vi "ReferenceGenerator_L.vi"(0 "Force_peak":sgl, 7 "Param In":T1, 11 "에러 출력":errorcluster) -> (4 "Force_Reference_L":sgl, 8 "Param out":T1, 15 "에러 출력 2":errorcluster caption="에러 출력")   [LabVIEW 2019]
uses:
  2c05c21f-2422-45a3-bbcb-ce1bef1032d3.vi
  7badd912-9f6d-4c0a-875e-7b5582638917.vi
panel:
  out "Force_mode_L":bool
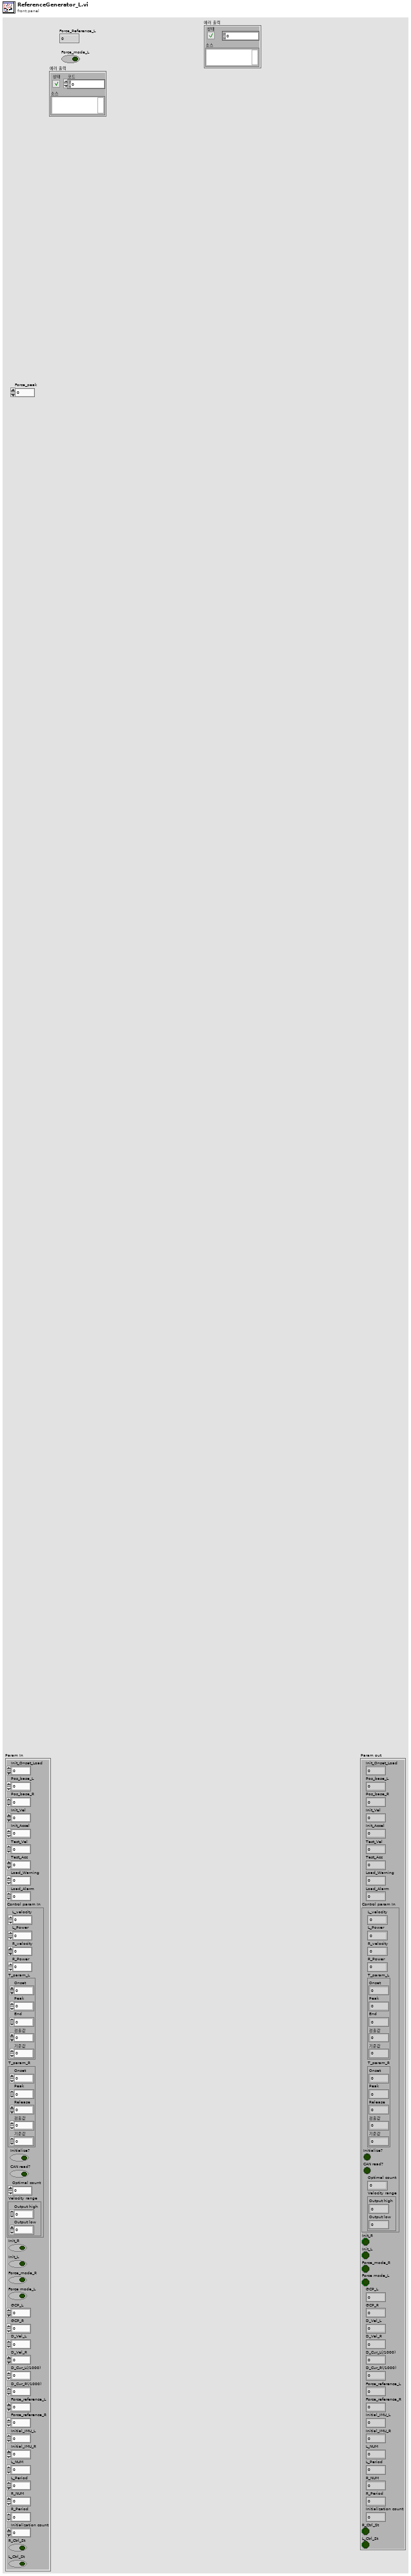
[diagram p1: front panel]
types:
  T1 = cluster{"Init_Onset_Load":sgl, "Pos_base_L":sgl, "Pos_base_R":sgl, "Init_Vel":i32, "Init_Accel":u32, "Test_Vel":i32, "Test_Acc":u32, "Load_Warning":sgl, "Load_Alarm":sgl, "Control param In":cluster{"L_velocity":u32, "L_Power":sgl, "R_velocity":u32, "R_Power":sgl, "T_param_L":cluster{"Onset":sgl, "Peak":sgl, "End":sgl, "검출값":sgl, "기준값":sgl}, "T_param_R":cluster{"Onset":sgl, "Peak":sgl, "Release":sgl, "검출값":sgl, "기준값":sgl}, "Initialize?":bool, "CAN read?":bool, "Optimal count":i32, "Velocity range":cluster{"Output high":dbl, "Output low":dbl}}, "Init_R":bool, "Init_L":bool, "Force_mode_R":bool, "Force mode_L":bool, "GCP_L":sgl, "GCP_R":sgl, "D_Vel_L":sgl, "D_Vel_R":sgl, "D_Cur_L(/1000)":sgl, "D_Cur_R(/1000)":sgl, "Force_reference_L":sgl, "Force_reference_R":sgl, "Initial_IMU_L":sgl, "Initial_IMU_R":sgl, "L_NUM":u32, "L_Period":i16, "R_NUM":u32, "R_Period":i16, "Initialization count":i32, "R_Ctrl_St":bool, "L_Ctrl_St":bool}
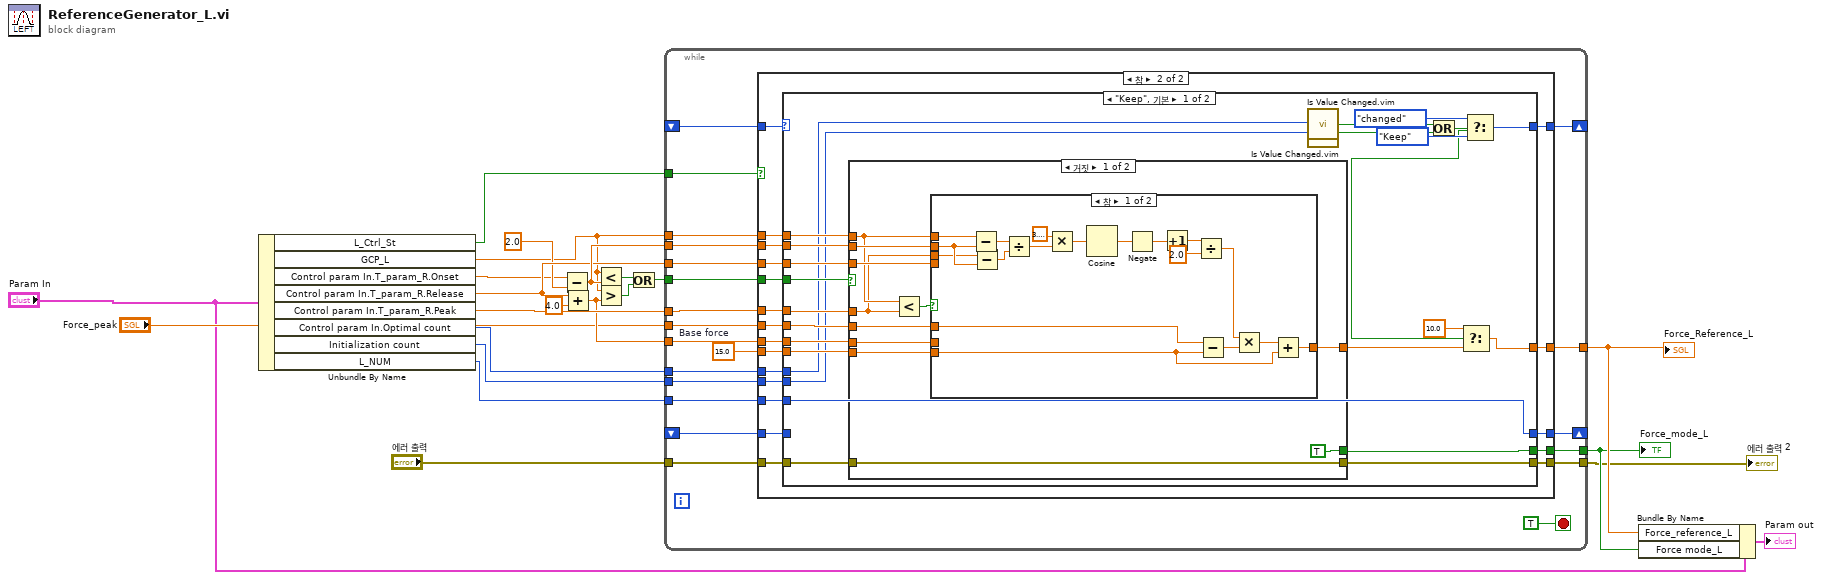
[diagram p0: block diagram]
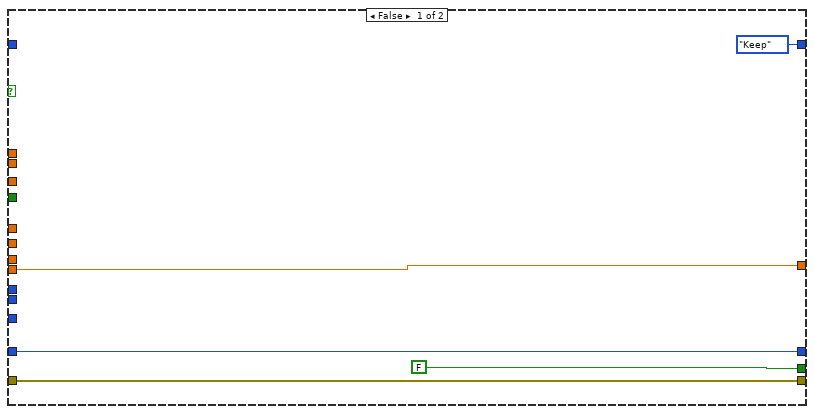
[diagram p2: hidden frame]
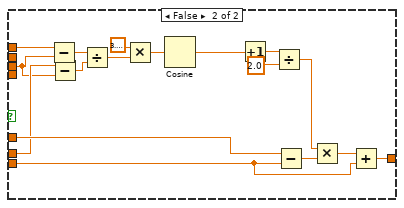
[diagram p3: hidden frame]
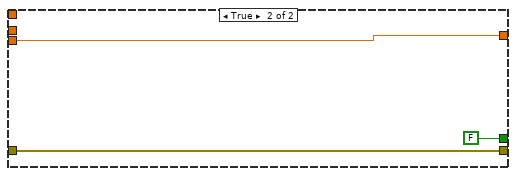
[diagram p4: hidden frame]
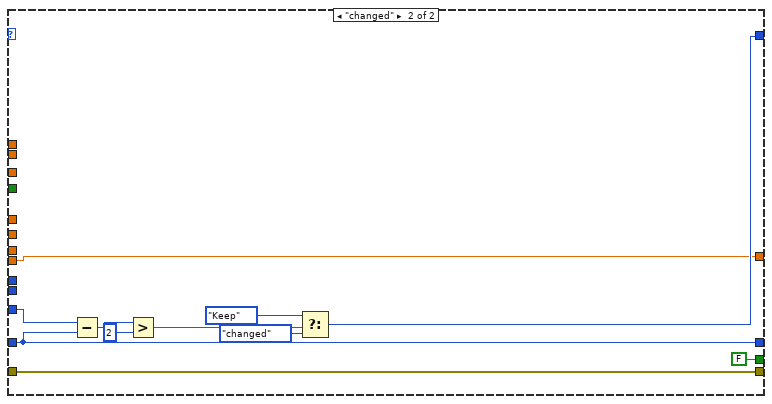
[diagram p5: hidden frame]
diagram:
  n1 = Unbundle By Name("Param In") -> ("L_Ctrl_St"=w2:bool, "GCP_L"=w4:sgl, "Control param In.T_param_R.Onset"=w13:sgl, "Control param In.T_param_R.Release"=w21:sgl, "Control param In.T_param_R.Peak"=w20:sgl, "Control param In.Optimal count"=w12:i32, "Initialization count"=w11:i32, "L_NUM"=w10:u32)
  n2 = Subtract(x=w13, y=sgl 2.0) -> (x-y=w22:sgl)
  n3 = Add(x=w21, y=sgl 4.0) -> (x+y=w19:sgl)
  n4 = Less?(x=w4, y=w22) -> (x < y?=w16:bool)
  n5 = Greater?(x=w4, y=w19) -> (0:w17:bool)
  n6 = Or(x=w16, y=w17) -> (x .or. y?=w18:bool)
  n7 = while {
    tunnel: w22 -> [w43]
    tunnel: w21 -> [w42]
    tunnel: w20 -> [w28]
    tunnel: w19 -> [w41]
    tunnel: w4 -> [w37]
    tunnel: w2 -> [w36]
    tunnel: "Force_peak" -> [w35]
    tunnel: [w32] -> w7
    tunnel: w12 -> [w31]
    tunnel: w11 -> [w30]
    tunnel: w10 -> [w29]
    tunnel: w18 -> [w40]
    tunnel: [w33] -> w6
    tunnel: "에러 출력" -> [w38]
    tunnel: [w34] -> w5
    shift-right: [w26] -> _
    shift-left: _ -> [w25]
    shift-right: [w24] -> _
    shift-left: _ -> [w23]
    stop <- TRUE stop-if-true
    w39 = sgl 15.0  # Base force
    n8 = case shown="참" w36 {
      tunnel: w43 -> [_ w67]
      tunnel: w42 -> [_ w66]
      tunnel: w41 -> [_ w65]
      tunnel: w40 -> [_ w57]
      tunnel: w37 -> [_ w64]
      tunnel: w35 -> [_ w63]
      tunnel: w39 -> [w48 w62]
      tunnel: w38 -> [w46 w61]
      tunnel: [w46 w60] -> w34
      tunnel: [FALSE w59] -> w33
      tunnel: [w48 w58] -> w32
      tunnel: w31 -> [_ w55]
      tunnel: w30 -> [_ w54]
      tunnel: w29 -> [_ w51]
      tunnel: w28 -> [_ w56]
      tunnel: [enum16{"Keep", "changed"}."Keep" w53] -> w26
      tunnel: w25 -> [_ w52]
      tunnel: [w44 w50] -> w24
      tunnel: w23 -> [w44 w49]
      frame False {
      }
      frame True {
        n9 = case shown="\"Keep\", 기본" w52 {
          tunnel: w67 -> [w90 _]
          tunnel: w66 -> [w89 _]
          tunnel: w65 -> [w88 _]
          tunnel: w64 -> [w87 _]
          tunnel: w63 -> [w86 _]
          tunnel: w62 -> [w85 w142]
          tunnel: w61 -> [w84 w140]
          tunnel: [w83 w140] -> w60
          tunnel: [w82 FALSE] -> w59
          tunnel: [w69 w142] -> w58
          tunnel: w57 -> [w81 _]
          tunnel: w56 -> [w80 _]
          tunnel: w55 -> [w76 _]
          tunnel: w54 -> [w75 _]
          tunnel: [w73 w144] -> w53
          tunnel: w51 -> [w68 w150]
          tunnel: [w68 w143] -> w50
          tunnel: w49 -> [_ w143]
          frame "Keep", Default {
            n10 = case shown="거짓" w81 {
              tunnel: w87 -> [w92 _]
              tunnel: w85 -> [w98 w138]
              tunnel: [TRUE FALSE] -> w82
              tunnel: [w93 w138] -> w71
              tunnel: w86 -> [w96 _]
              tunnel: w88 -> [w99 _]
              tunnel: w90 -> [w100 _]
              tunnel: w84 -> [w95 w137]
              tunnel: [w95 w137] -> w83
              tunnel: w89 -> [w94 _]
              tunnel: w80 -> [w91 _]
              frame False {
                n11 = Less?(x=w92, y=w91) -> (x < y?=w101:bool)
                n12 = case shown="참" w101 {
                  tunnel: w92 -> [w119 w122]
                  tunnel: w100 -> [w118 _]
                  tunnel: w91 -> [w102 w121]
                  tunnel: w99 -> [_ w123]
                  tunnel: w98 -> [w105 w126]
                  tunnel: [w104 w125] -> w93
                  tunnel: w96 -> [w103 w124]
                  tunnel: w94 -> [_ _]
                  frame True {
                    n13 = Subtract(x=w119, y=w118) -> (x-y=w117:sgl)
                    n14 = Subtract(x=w102, y=w118) -> (x-y=w116:sgl)
                    n15 = Divide(x=w117, y=w116) -> (x/y=w115:sgl)
                    n16 = Multiply(x=3.141592653589793, y=w115) -> (x*y=w113:dbl)
                    n17 = Cosine(x=w113) -> (cos(x)=w112:dbl)
                    n18 = Negate(x=w112) -> (-x=w111:dbl)
                    n19 = Increment(x=w111) -> (x+1=w110:dbl)
                    n20 = Divide(x=w110, y=2.0) -> (x/y=w107:dbl)
                    n21 = Subtract(x=w103, y=w105) -> (x-y=w108:sgl)
                    n22 = Multiply(x=w107, y=w108) -> (x*y=w106:dbl)
                    n23 = Add(x=w106, y=w105) -> (x+y=w104:dbl)
                  }
                  frame False {
                    n24 = Subtract(x=w122, y=w121) -> (x-y=w136:sgl)
                    n25 = Subtract(x=w123, y=w121) -> (x-y=w135:sgl)
                    n26 = Divide(x=w136, y=w135) -> (x/y=w134:sgl)
                    n27 = Multiply(x=3.141592653589793, y=w134) -> (x*y=w132:dbl)
                    n28 = Cosine(x=w132) -> (cos(x)=w120:dbl)
                    n29 = Increment(x=w120) -> (x+1=w131:dbl)
                    n30 = Divide(x=w131, y=2.0) -> (x/y=w128:dbl)
                    n31 = Subtract(x=w124, y=w126) -> (x-y=w129:sgl)
                    n32 = Multiply(x=w128, y=w129) -> (x*y=w127:dbl)
                    n33 = Add(x=w127, y=w126) -> (x+y=w125:dbl)
                  }
                }
              }
              frame True {
              }
            }
            n34 = call "Is Value Changed.vim"("value"=w76) -> ("changed or first call?"=w78:bool)
            n35 = call "Is Value Changed.vim"("value"=w75) -> ("changed or first call?"=w79:bool)
            n36 = Or(x=w78, y=w79) -> (x .or. y?=w72:bool)
            n37 = Select(t=10.0, s=w72, f=w71) -> (s? t:f=w69:dbl)
            n38 = Select(t=enum16{"Keep", "changed"}."changed", s=w72, f=enum16{"Keep", "changed"}."Keep") -> (s? t:f=w73:enum16{"Keep", "changed"})
          }
          frame "changed" {
            n39 = Subtract(x=w150, y=w143) -> (x-y=w149:u32)
            n40 = Greater?(x=w149, y=u32 2) -> (0:w145:bool)
            n41 = Select(t=enum16{"Keep", "changed"}."Keep", s=w145, f=enum16{"Keep", "changed"}."changed") -> (s? t:f=w144:enum16{"Keep", "changed"})
          }
        }
      }
    }
  }
  "Force_mode_L" <- w6
  "Force_Reference_L" <- w7
  "에러 출력 2" <- w5
  n42 = Bundle By Name(cluster="Param In", "Force_reference_L"=w7, "Force mode_L"=w6) -> (→"Param out":T1)
